vi "Main_10b refactor.vi"() -> ()   [LabVIEW 2020]
panel:
  out "Final X":i32
  out "Values of that cycle":i32[](array[numeric])
  in  "Example 2":string="addx 15\naddx -11\naddx 6\naddx -3\naddx 5\naddx -1\naddx -8\naddx 13\naddx 4\nnoop\naddx -1\naddx 5\naddx -1\naddx 5\naddx -1\naddx 5\naddx -1\naddx 5\naddx -1\naddx -35\naddx 1\naddx 24\naddx -19\naddx 1\naddx 16\naddx -11\nnoop\nnoop\naddx 21\naddx -15\nnoop\nnoop\naddx -3\naddx 9\naddx 1\naddx -3\naddx 8\naddx 1\naddx 5\nnoop\nnoop\nnoop\nnoop\nnoop\naddx -36\nnoop\naddx 1\naddx 7\nnoop\nnoop\nnoop\naddx 2\naddx 6\nnoop\nnoop\nnoop\nnoop\nnoop\naddx 1\nnoop\nnoop\naddx 7\naddx 1\nnoop\naddx -13\naddx 13\naddx 7\nnoop\naddx 1\naddx -33\nnoop\nnoop\nnoop\naddx 2\nnoop\nnoop\nnoop\naddx 8\nnoop\naddx -1\naddx 2\naddx 1\nnoop\naddx 17\naddx -9\naddx 1\naddx 1\naddx -3\naddx 11\nnoop\nnoop\naddx 1\nnoop\naddx 1\nnoop\nnoop\naddx -13\naddx -19\naddx 1\naddx 3\naddx 26\naddx -30\naddx 12\naddx -1\naddx 3\naddx 1\nnoop\nnoop\nnoop\naddx -9\naddx 18\naddx 1\naddx 2\nnoop\nnoop\naddx 9\nnoop\nnoop\nnoop\naddx -1\naddx 2\naddx -37\naddx 1\naddx 3\nnoop\naddx 15\naddx -21\naddx 22\naddx -6\naddx 1\nnoop\naddx 2\naddx 1\nnoop\naddx -10\nnoop\nnoop\naddx 20\naddx 1\naddx 2\naddx 2\naddx -6\naddx -11\nnoop\nnoop\nnoop"
  out "sum":i32
  in  "Puzzle":string="addx 1\naddx 5\nnoop\naddx -1\nnoop\naddx 3\naddx 29\naddx -1\naddx -21\naddx 5\nnoop\naddx -20\naddx 21\naddx 2\naddx 8\naddx -1\nnoop\nnoop\nnoop\nnoop\naddx 6\naddx -1\naddx -37\naddx 40\naddx -10\naddx -25\naddx 5\naddx 2\naddx 5\nnoop\nnoop\nnoop\naddx 21\naddx -20\naddx 2\nnoop\naddx 3\naddx 2\naddx -5\naddx 12\naddx 3\nnoop\naddx 2\naddx 3\naddx -2\naddx -37\naddx 1\naddx 5\naddx 3\naddx -2\naddx 2\naddx 29\naddx -22\naddx 13\nnoop\naddx -8\naddx -6\naddx 7\naddx 2\nnoop\naddx 7\naddx -2\naddx 5\naddx 2\naddx -26\naddx -11\nnoop\nnoop\naddx 6\naddx 1\naddx 1\nnoop\naddx 4\naddx 5\nnoop\nnoop\naddx -2\naddx 3\nnoop\naddx 2\naddx 5\naddx 2\naddx -22\naddx 27\naddx -1\naddx 1\naddx 5\naddx 2\nnoop\naddx -39\naddx 22\nnoop\naddx -15\naddx 3\naddx -2\naddx 2\naddx -2\naddx 9\naddx 3\nnoop\naddx 2\naddx 3\naddx -2\naddx 2\nnoop\nnoop\nnoop\naddx 5\naddx -17\naddx 24\naddx -7\naddx 8\naddx -36\naddx 2\naddx 3\naddx 33\naddx -32\naddx 4\naddx 1\nnoop\naddx 5\nnoop\nnoop\naddx 20\naddx -15\naddx 4\nnoop\naddx 1\nnoop\naddx 4\naddx 6\naddx -30\naddx 30\nnoop\nnoop\nnoop\nnoop\nnoop"
  in  "Example":string="noop\naddx 3\naddx -5"
  out "Screen":bool[][](array[boolean])
  # "EALGULPG"
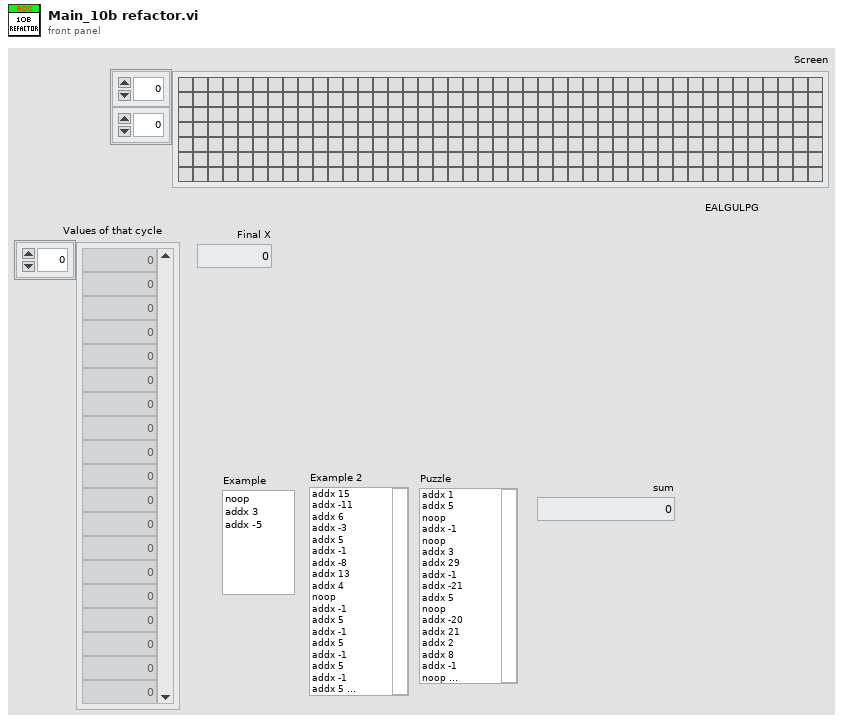
[diagram p1: front panel]
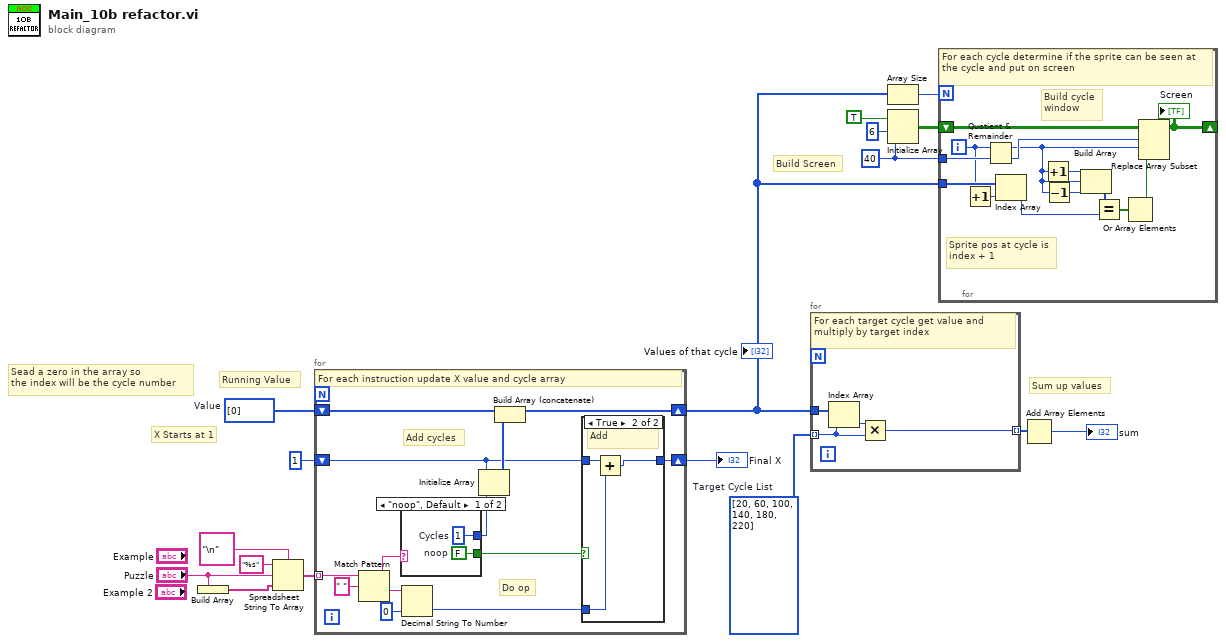
[diagram p0: block diagram]
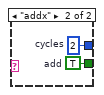
[diagram p2: hidden frame]
diagram:
  w5 = i32[] [20, 60, 100, 140, 180, 220]  # Target Cycle List
  w9 = i32[] [0]  # Value
  w13 = 40 ("dimension size")
  # "Build Screen"
  # "Sum up values"
  # "Sead a zero in the array so\nthe index will be the cycle number"
  # "X Starts at 1"
  # "Running Value"
  n1 = Build Array("Puzzle") -> (w7:string[])
  n2 = Spreadsheet String To Array(delimiter (Tab)="\n", format string="%s", spreadsheet string="Puzzle", array type (2D Dbl)=w7) -> (array=w8:string[])
  n3 = for {
    shift-right: [w26] -> w6
    shift-left: 1 -> [w28]
    shift-right: [w27] -> w1
    shift-left: w9 -> [w30]
    tunnel: w8 -> [w25] mode=indexing
    # "Do op"
    # "Add cycles"
    # "For each instruction update X value and cycle array"
    n4 = Match Pattern(string=w25, regular expression=" ") -> (before substring=w20:string, after substring=w24:string)  [unwired: 1 in, 2 out]
    n5 = case shown="\"noop\", Default" w20 {
      tunnel: [w32 w34] -> w19
      tunnel: [w31 w33] -> w18
      frame "noop", Default {
        w31 = FALSE  # noop
        w32 = 1  # Cycles
      }
      frame "addx" {
        w33 = TRUE  # add
        w34 = 2  # cycles
      }
    }
    n6 = Decimal String To Number(string=w24, default (0L)=0 ("default (0 I32)")) -> (number=w21:i32)  [unwired: 1 in, 1 out]
    n7 = Initialize Array(w28, w19) -> (w29:i32[])
    n8 = Build Array (concatenate)(w30, w29) -> (w27:i32[])
    n9 = case shown="True" w18 {
      tunnel: w28 -> [w35 w38]
      tunnel: w21 -> [_ w37]
      tunnel: [w35 w36] -> w26
      frame False {
        # "noop"
      }
      frame True {
        # "Add"
        n10 = Add(x=w38, y=w37) -> (x+y=w36:i32)
      }
    }
  }
  "Values of that cycle" <- w1
  "Final X" <- w6
  n11 = for {
    tunnel: w5 -> [w40] mode=indexing
    tunnel: w1 -> [w42]
    tunnel: [w39] -> w4 mode=indexing
    # "For each target cycle get value and multiply by target index"
    n12 = Index Array(array=w42, index=w40) -> (element=w41:i32)
    n13 = Multiply(x=w41, y=w40) -> (x*y=w39:i32)
  }
  n14 = Array Size(array=w1) -> (size(s)=w14:i32)
  n15 = Initialize Array(TRUE ("Boolean"), 6 ("dimension size"), w13) -> (w15:bool[][])
  n16 = for {
    N: w14 -> [_]
    tunnel: w1 -> [w46]
    shift-right: [w55] -> _
    shift-left: w15 -> [w56]
    tunnel: w13 -> [w45]
    i -> [w44]
    # "Build cycle\nwindow"
    # "Sprite pos at cycle is\nindex + 1"
    # "For each cycle determine if the sprite can be seen at the cycle and put on screen"
    n17 = Increment(x=w44) -> (x+1=w48:i32)
    n18 = Quotient & Remainder(x=w44, y=w45) -> (x-y*floor(x/y)=w43:i32, floor(x/y)=w50:i32)
    n19 = Index Array(array=w46, index=w48) -> (element=w47:i32)
    n20 = Increment(x=w43) -> (x+1=w54:i32)
    n21 = Decrement(x=w43) -> (x-1=w53:i32)
    n22 = Build Array(w54, w43, w53) -> (w52:i32[])
    n23 = Equal?(x=w52, y=w47) -> (x = y?=w51:bool[])
    n24 = Or Array Elements(Boolean array=w51) -> (logical OR=w49:bool)
    n25 = Replace Array Subset(array=w56, new element=w49, index (row)=w50, index (col)=w43) -> (w55:bool[][])
    "Screen" <- w55
  }
  n26 = Add Array Elements(numeric array=w4) -> (sum=→"sum":i32)
